vi "daq_bandstop.vi"() -> ()   [LabVIEW 2023]
uses:
  <vilib>/addons/Biomedical/Biosignal Measurements/EEG/EEG FFT Spectrum (Waveform).vi
  <vilib>/addons/Biomedical/NI_BMTK_Measurements.lvlib
panel:
  out "Gamma Wave FFT Spectrum":cluster{"f0":dbl, "df":dbl, "S(f)":dbl[]}(graph)
  out "Beta Wave FFT Spectrum":cluster{"f0":dbl, "df":dbl, "S(f)":dbl[]}(graph)
  out "Alpha Wave FFT Spectrum":cluster{"f0":dbl, "df":dbl, "S(f)":dbl[]}(graph)
  out "Theta Wave FFT Spectrum":cluster{"f0":dbl, "df":dbl, "S(f)":dbl[]}(graph)
  out "Delta Wave FFT Spectrum":cluster{"f0":dbl, "df":dbl, "S(f)":dbl[]}(graph)
  out "EEG FFT Spectrum":cluster{"f0":dbl, "df":dbl, "S(f)":dbl[]}(graph)
  out "Delta Wave":dynamicdata(graph)
  out "Gamma Wave":dynamicdata(graph)
  out "Beta Wave":dynamicdata(graph)
  out "Alpha Wave":dynamicdata(graph)
  out "Theta Wave":dynamicdata(graph)
  out "EEG Signal":dynamicdata(graph)
  in  "stop":bool
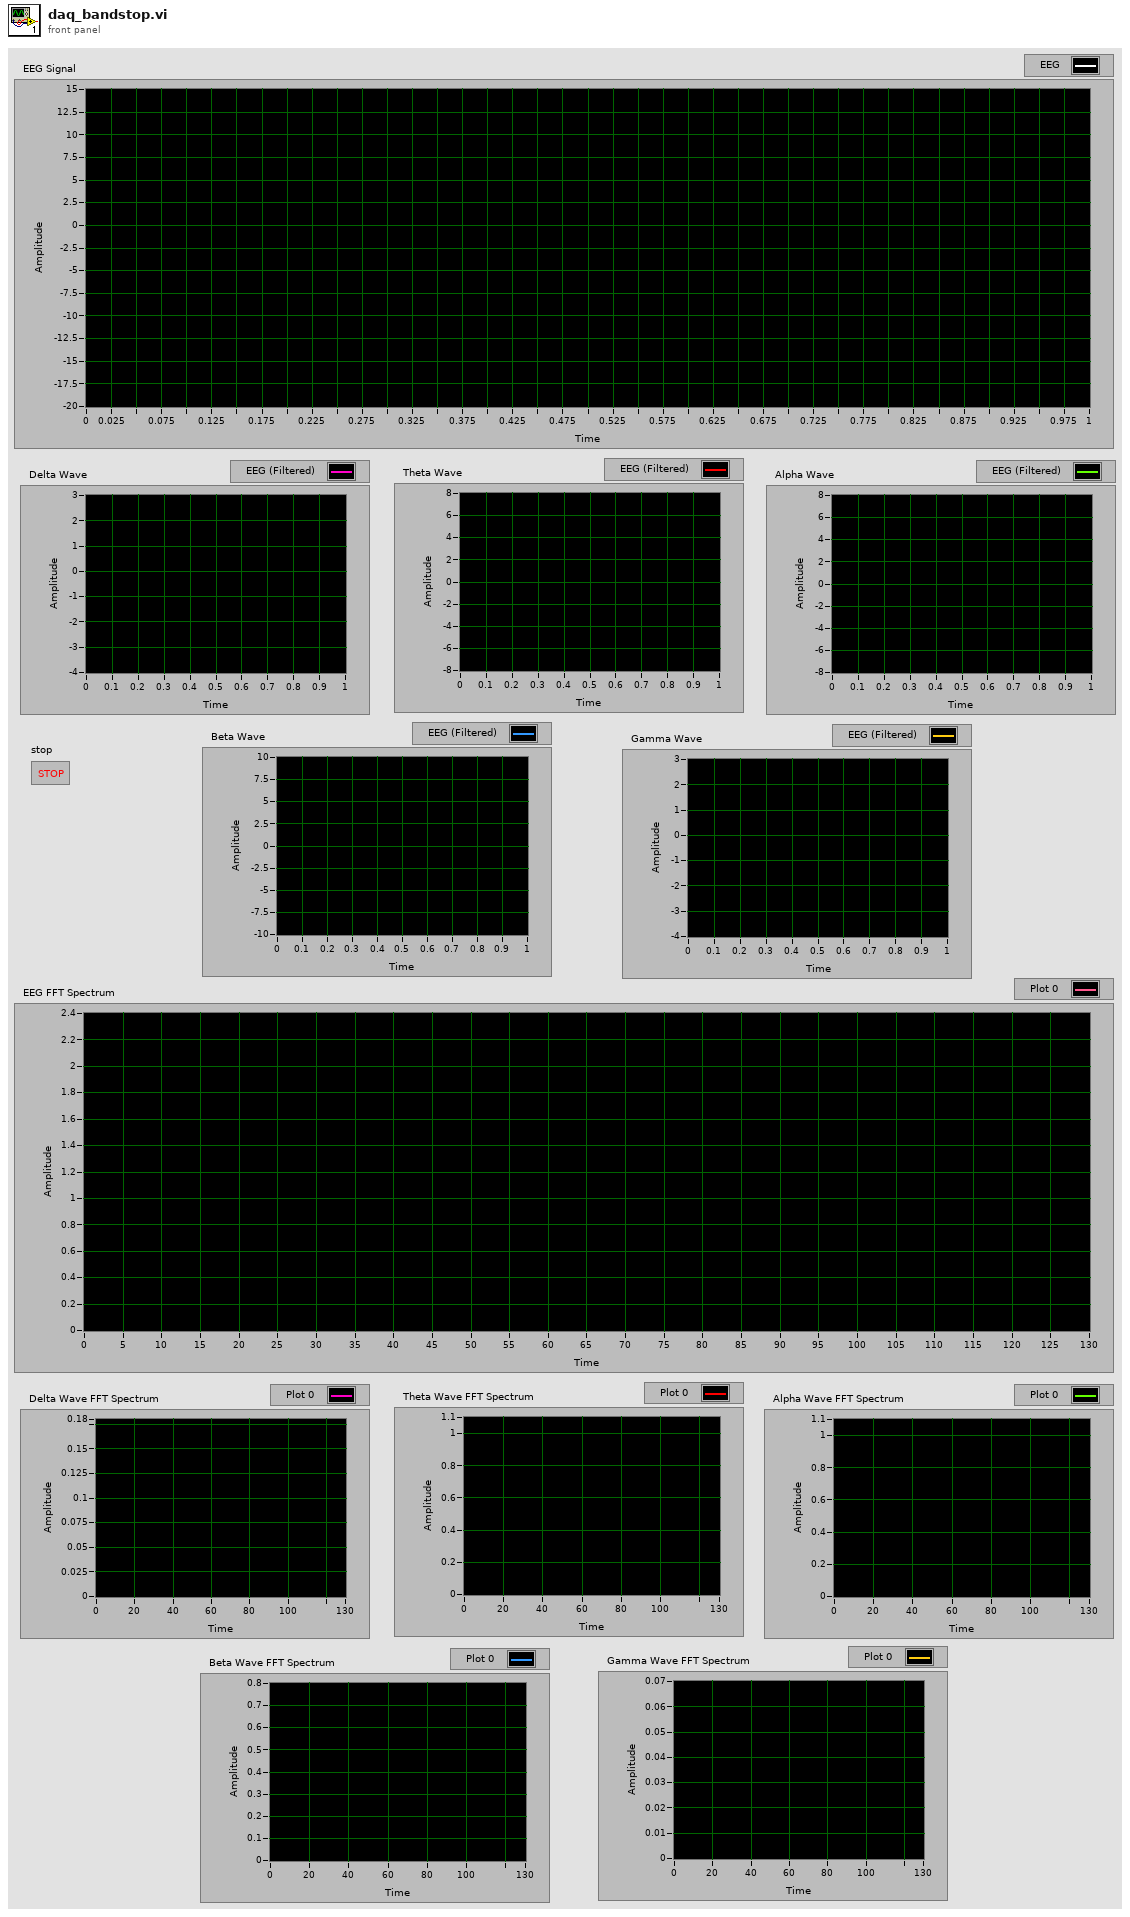
[diagram p1: front panel]
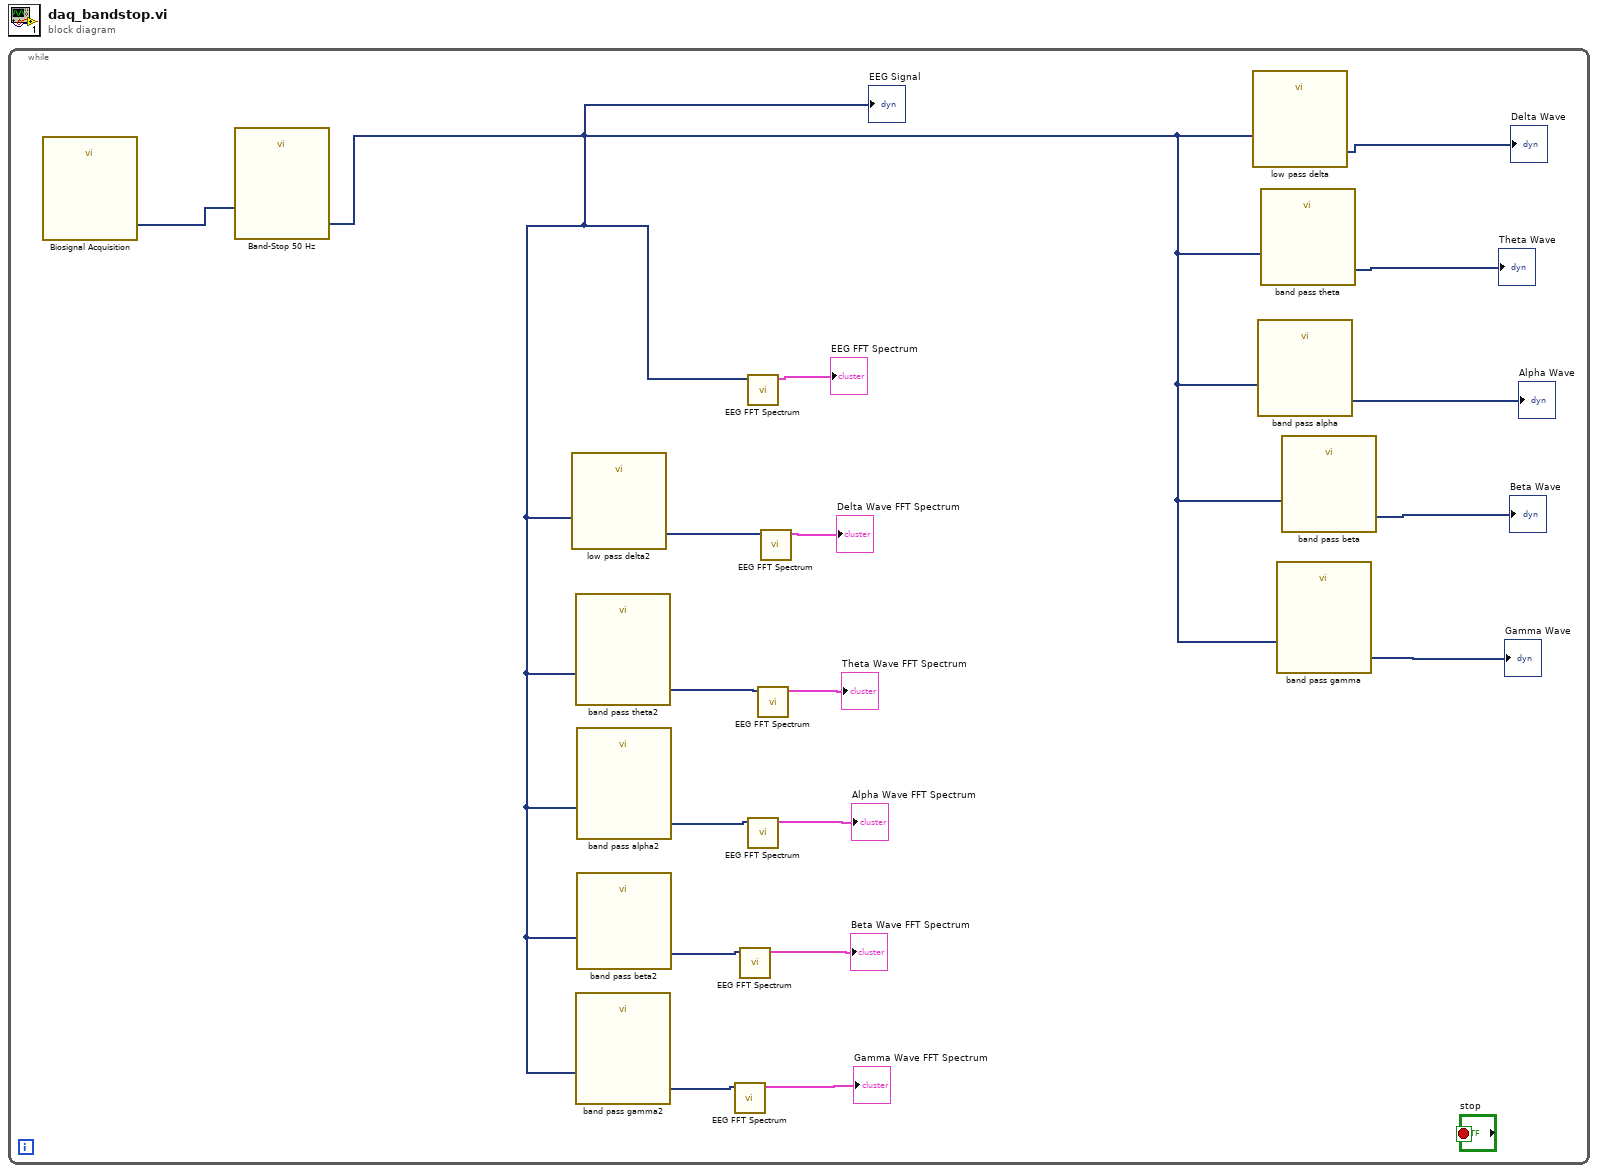
[diagram p0: block diagram]
diagram:
  n1 = while {
    stop <- "stop" stop-if-true
    n2 = call "Biosignal Acquisition"() -> ("biosignal"=w2:dynamicdata)  [unwired: 10 in, 1 out]
    n3 = call "Band-Stop 50 Hz"("Signal"=w2) -> ("Filtered Signal"=w1:dynamicdata)  [unwired: 9 in, 1 out]
    "EEG Signal" <- w1
    n4 = call "low pass delta2"("Signal"=w1) -> ("Filtered Signal"=w11:dynamicdata)  [unwired: 9 in, 1 out]
    n5 = call "band pass theta2"("Signal"=w1) -> ("Filtered Signal"=w10:dynamicdata)  [unwired: 9 in, 1 out]
    n6 = call "band pass gamma2"("Signal"=w1) -> ("Filtered Signal"=w3:dynamicdata)  [unwired: 9 in, 1 out]
    n7 = call "band pass alpha2"("Signal"=w1) -> ("Filtered Signal"=w7:dynamicdata)  [unwired: 9 in, 1 out]
    n8 = call "band pass beta2"("Signal"=w1) -> ("Filtered Signal"=w5:dynamicdata)  [unwired: 9 in, 1 out]
    n9 = call-poly <vilib>:"EEG FFT Spectrum.vi"("EEG"=w3) -> ("FFT spectrum"=→"Gamma Wave FFT Spectrum":cluster{"f0":dbl, "df":dbl, "S(f)":dbl[]})  [unwired: 8 in, 2 out]
    n10 = call-poly <vilib>:"EEG FFT Spectrum.vi"("EEG"=w5) -> ("FFT spectrum"=→"Beta Wave FFT Spectrum":cluster{"f0":dbl, "df":dbl, "S(f)":dbl[]})  [unwired: 8 in, 2 out]
    n11 = call-poly <vilib>:"EEG FFT Spectrum.vi"("EEG"=w1) -> ("FFT spectrum"=→"EEG FFT Spectrum":cluster{"f0":dbl, "df":dbl, "S(f)":dbl[]})  [unwired: 8 in, 2 out]
    n12 = call-poly <vilib>:"EEG FFT Spectrum.vi"("EEG"=w7) -> ("FFT spectrum"=→"Alpha Wave FFT Spectrum":cluster{"f0":dbl, "df":dbl, "S(f)":dbl[]})  [unwired: 8 in, 2 out]
    n13 = call-poly <vilib>:"EEG FFT Spectrum.vi"("EEG"=w10) -> ("FFT spectrum"=→"Theta Wave FFT Spectrum":cluster{"f0":dbl, "df":dbl, "S(f)":dbl[]})  [unwired: 8 in, 2 out]
    n14 = call-poly <vilib>:"EEG FFT Spectrum.vi"("EEG"=w11) -> ("FFT spectrum"=→"Delta Wave FFT Spectrum":cluster{"f0":dbl, "df":dbl, "S(f)":dbl[]})  [unwired: 8 in, 2 out]
    n15 = call "low pass delta"("Signal"=w1) -> ("Filtered Signal"=→"Delta Wave":dynamicdata)  [unwired: 9 in, 1 out]
    n16 = call "band pass alpha"("Signal"=w1) -> ("Filtered Signal"=→"Alpha Wave":dynamicdata)  [unwired: 9 in, 1 out]
    n17 = call "band pass theta"("Signal"=w1) -> ("Filtered Signal"=→"Theta Wave":dynamicdata)  [unwired: 9 in, 1 out]
    n18 = call "band pass gamma"("Signal"=w1) -> ("Filtered Signal"=→"Gamma Wave":dynamicdata)  [unwired: 9 in, 1 out]
    n19 = call "band pass beta"("Signal"=w1) -> ("Filtered Signal"=→"Beta Wave":dynamicdata)  [unwired: 9 in, 1 out]
  }
